vi "Simple Reader.vi"(8 "error in (no error)":errorcluster, 11 "Prema Driver in":refnum<class "Prema Driver.lvclass">) -> (0 "error out":errorcluster, 2 "Signals":dbl[](array[numeric]), 3 "Prema Driver out":refnum<class "Prema Driver.lvclass">)   [LabVIEW 2021, in "Prema Driver.lvclass"]
uses:
  Prema Driver.lvclass
  C:/Git/NHMFL_Core/Libraries/Instruments/VISA Instrument/VISA Instrument.lvclass
  VISA Instrument/VISA Instrument.lvclass/VISA Instrument.ctl
  VISA Instrument/Read VISA resource.vi
  VISA Instrument/Write VISA resource.vi
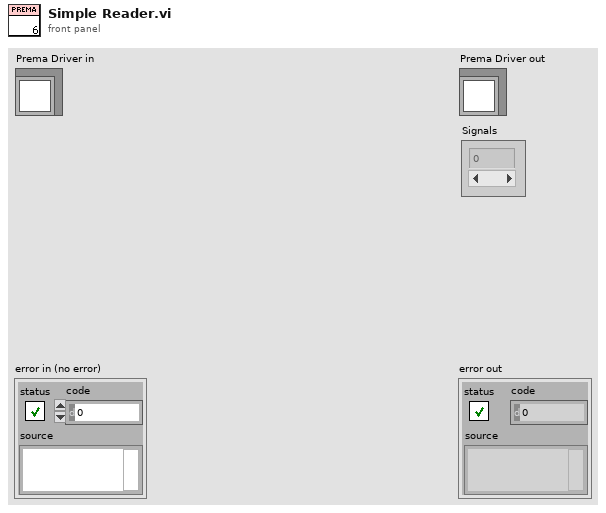
[diagram p1: front panel]
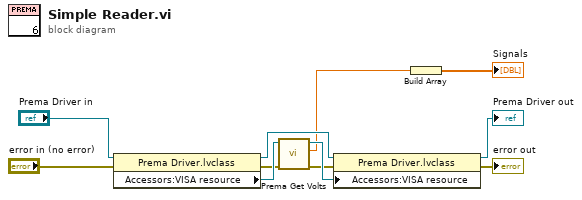
[diagram p0: block diagram]
diagram:
  n1 = property class="Prema Driver.lvclass"(reference="Prema Driver in", error in="error in (no error)") -> (reference out=w8:refnum<class "Prema Driver.lvclass">, error out=w2:errorcluster, "Accessors:VISA resource"=w9:refnum<visa-resource-name>)
  n2 = call "Prema Get Volts.vi"("error in"=w2, "VISA resource name"=w9) -> ("error out"=w1:errorcluster, "value"=w4:dbl, "VISA resource name out"=w7:refnum<visa-resource-name>)  [unwired: 6 in, 1 out]
  n3 = property class="Prema Driver.lvclass"(reference=w8, error in=w1, "Accessors:VISA resource"=w7) -> (reference out=→"Prema Driver out":refnum<class "Prema Driver.lvclass">, error out=→"error out":errorcluster)
  n4 = Build Array(w4) -> (→"Signals":dbl[])
